vi "Boolean to Yes-No string.vi"(1 "Boolean":bool) -> (0 "Yes No":string)   [LabVIEW 2013, in "Strings Lib.lvlib"]
uses:
  Strings Lib.lvlib
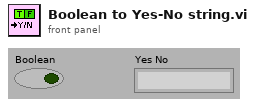
[diagram p1: front panel]
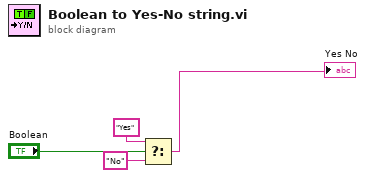
[diagram p0: block diagram]
diagram:
  n1 = Select(t="Yes" ("element"), s="Boolean", f="No") -> (s? t:f=→"Yes No":string)
